vi "General LS Linear Fit PtByPt.vi"(0 "H":dbl[](array[numeric]), 1 "initialize":bool, 5 "y":dbl format="%0.2f", 7 "Standard Deviation":dbl[](array[numeric]), 9 "covariance selector":T1(ring), 11 "algorithm":T2(ring), 12 "sample length":i32=100) -> (4 "Coefficients":dbl[](array[numeric]), 6 "Best Fit":dbl[](array[numeric]), 8 "Covariance":dbl[][](array[numeric]), 10 "mse":dbl format="%0.2f", 15 "error":i32)   [LabVIEW 2017, in "NI_PtbyPt.lvlib"]
doc: "Finds the <B>Best Fit</B> k-dimensional plane and the set of linear coefficients for the set of input data points specified by <B>sample length</B>."
uses:
  <vilib>/ptbypt/NI_PtbyPt.lvlib
  <vilib>/Analysis/NI_AALPro.lvlib
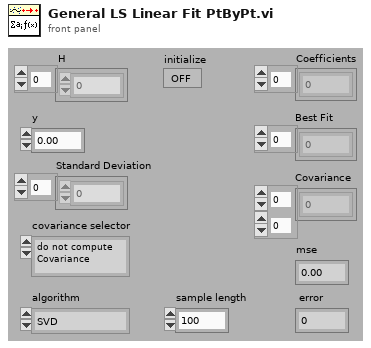
[diagram p1: front panel]
types:
  T1 = enum16{"do not compute Covariance", " compute Covariance"}
  T2 = enum32{"SVD", "Givens", "Givens2", "Householder", "LU Decomposition", "Cholesky"}
  T3 = typedef "NI_Matrix.lvlib/RealMatrix.ctl" = dbl[][]
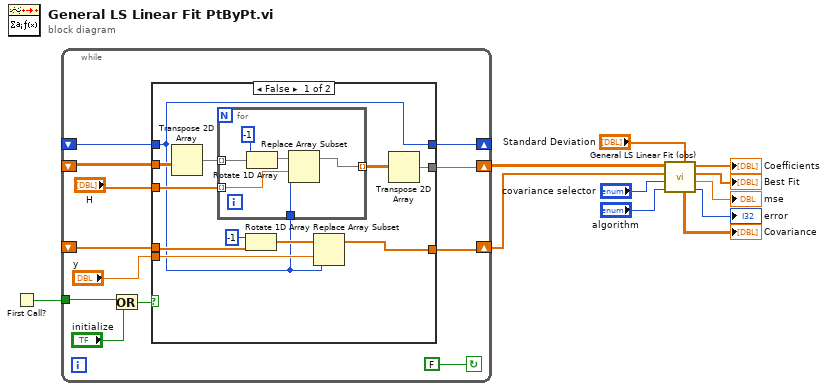
[diagram p0: block diagram]
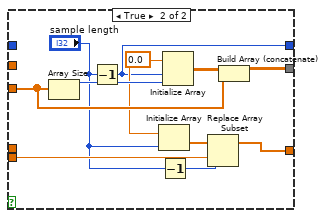
[diagram p2: hidden frame]
diagram:
  n1 = First Call?() -> (First Call?: T/F=w11:bool)
  n2 = while {
    shift-left: _ -> [w12]
    shift-right: [w13] -> _
    tunnel: w11 -> [w15]
    shift-left: _ -> [w18]
    shift-right: [w19] -> w8
    shift-left: _ -> [w23]
    shift-right: [w22] -> w9
    stop <- FALSE continue-if-true
    n3 = Or(x=w15, y="initialize") -> (x .or. y?=w14:bool)
    n4 = case shown="False" w14 {
      tunnel: w23 -> [w34 _]
      tunnel: [w31 w47] -> w22
      tunnel: "H" -> [w30 w45]
      tunnel: "y" -> [w26 w50]
      tunnel: [w25 w48] -> w19
      tunnel: w18 -> [w27 _]
      tunnel: [w24 w42] -> w13
      tunnel: w12 -> [w24 _]
      frame False {
        n5 = Transpose 2D Array(2D array=w34) -> (transposed array=w33:dbl[][])
        n6 = for {
          tunnel: w33 -> [w40] mode=indexing
          tunnel: w30 -> [w37] mode=indexing
          tunnel: [w36] -> w32 mode=indexing
          tunnel: w24 -> [w35]
          n7 = Rotate 1D Array(1:w40, 2:i16 -1 ("n")) -> (0:w38:dbl[])
          n8 = Replace Array Subset(array=w38, new element=w37, index=w35) -> (w36:dbl[])
        }
        n9 = Rotate 1D Array(1:w27, 2:i16 -1 ("n")) -> (0:w28:dbl[])
        n10 = Replace Array Subset(array=w28, new element=w26, index=w24) -> (w25:dbl[])
        n11 = Transpose 2D Array(2D array=w32) -> (transposed array=w31:dbl[][])
      }
      frame True {
        w43 = 0.0 ("Element Data")
        n12 = Array Size(array=w45) -> (size(s)=w46:i32)
        n13 = Decrement(x="sample length") -> (x-1=w42:i32)
        n14 = Initialize Array(w43, "sample length") -> (w51:dbl[])
        n15 = Decrement(x="sample length") -> (x-1=w49:i32)
        n16 = Initialize Array(w43, w42, w46) -> (w44:dbl[][])
        n17 = Replace Array Subset(array=w51, new element=w50, index=w49) -> (w48:dbl[])
        n18 = Build Array (concatenate)(w44, w45) -> (w47:dbl[][])
      }
    }
  }
  n19 = call <vilib>:"General LS Linear Fit (obs).vi"("H"=w9, "Y"=w8, "covariance selector"="covariance selector", "algorithm"="algorithm", "Standard Deviation"="Standard Deviation") -> ("Covariance"=→"Covariance":T3, "Coefficients"=→"Coefficients":dbl[], "Best Fit"=→"Best Fit":dbl[], "mse"=→"mse":dbl, "error"=→"error":i32)
